vi "Compare ni-xnet port with monitoring port.vi"(8 "Error In":errorcluster, 10 "NI-XNET Port Item Ref In":T1 format="%.0x", 11 "CD Port Item Ref In":T1 format="%.0x") -> (0 "Error Out":errorcluster, 2 "NI-XNET Port Item Ref Out":T1 format="%.0x", 3 "CD Port Item Ref Out":T1=18446744073709551615 format="%.0x")   [LabVIEW 2018, in "NI-XNET Monitor System Explorer.lvlib"]
uses:
  NI-XNET Monitor System Explorer.lvlib
  <vilib>/NI Veristand/Custom Device API/Custom Device Item Ref.ctl
  Shared/Constants.vi
  <vilib>/NI Veristand/Custom Device API/Get Item Property (Boolean).vi
  <vilib>/NI Veristand/Custom Device API/Get Item Property (String).vi
  <vilib>/NI Veristand/Custom Device API/Set Item Property (String).vi
  <vilib>/NI Veristand/Custom Device API/Custom Device API.lvlib
  Shared/NI-XNET Monitor Shared.lvlib
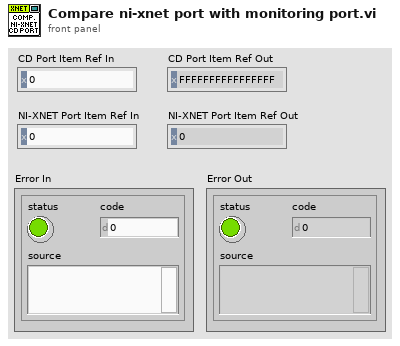
[diagram p1: front panel]
types:
  T1 = typedef "Custom Device API.lvlib/Custom Device Item Ref.ctl" = u64
  T2 = typedef "Custom Device API.lvlib/Custom Device Item Info.ctl" = cluster{"Name":string, "Is Channel":bool, "GUID":string, "Is Waveform":bool}
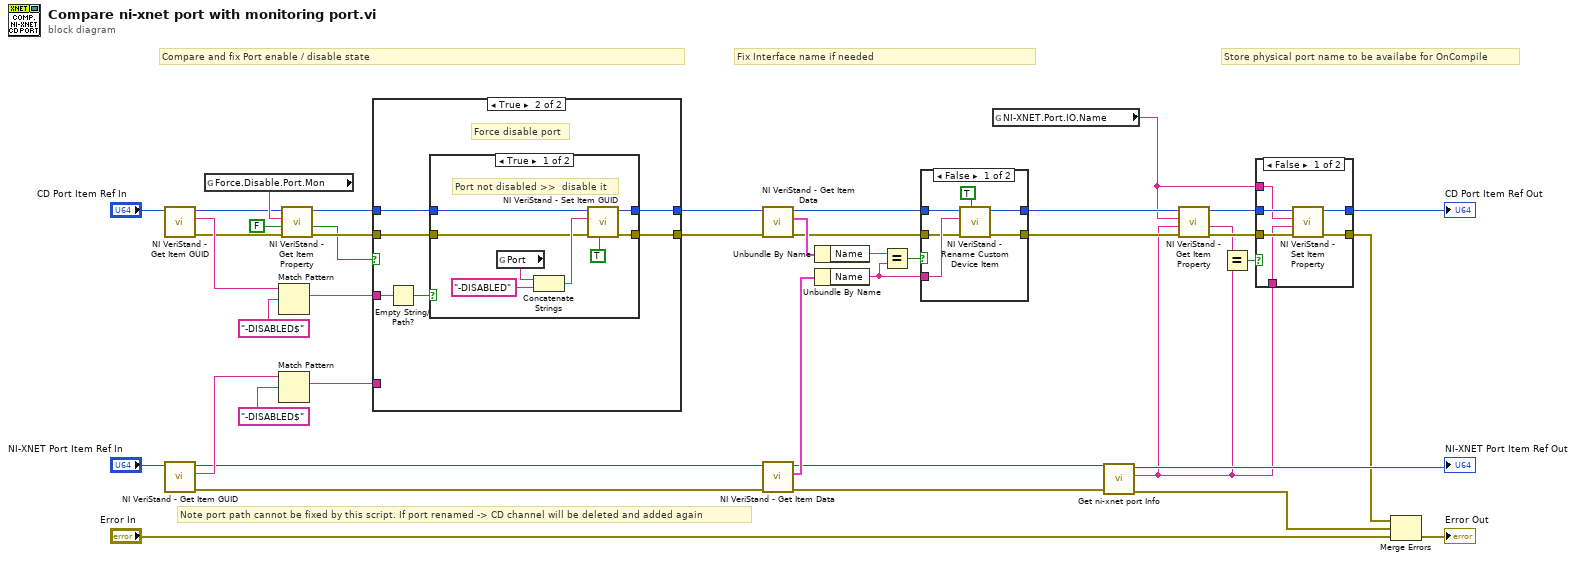
[diagram p0: block diagram]
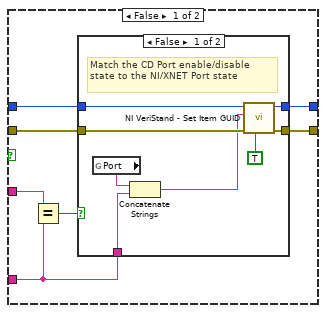
[diagram p4: hidden frame]
diagram:
  # "Note port path cannot be fixed by this script. If port renamed -> CD channel will be deleted and added again"
  # "Store physical port name to be availabe for OnCompile"
  # "Fix Interface name if needed"
  # "Compare and fix Port enable / disable state"
  n1 = call <vilib>:"NI VeriStand - Get Item GUID.vi"("Item Ref in"="CD Port Item Ref In") -> ("error out"=w33:errorcluster, "GUID"=w34:string, "Item Ref out"=w35:T1)  [unwired: 8 in]
  n2 = call <vilib>:"NI VeriStand - Get Item GUID.vi"("Item Ref in"="NI-XNET Port Item Ref In") -> ("error out"=w15:errorcluster, "GUID"=w32:string, "Item Ref out"=w31:T1)  [unwired: 8 in]
  n3 = global read "Constants.vi" "Force.Disable.Port.Mon"() -> (w39:string)
  n4 = Match Pattern(string=w34, regular expression="-DISABLED$") -> (match substring=w19:string)  [unwired: 1 in, 3 out]
  n5 = Match Pattern(string=w32, regular expression="-DISABLED$") -> (match substring=w20:string)  [unwired: 1 in, 3 out]
  n6 = call-poly <vilib>:"NI VeriStand - Get Item Property.vi"("error in (no error)"=w33, "Default Value"=FALSE, "Property Name"=w39, "Item Ref in"=w35) -> ("error out"=w36:errorcluster, "Value"=w16:bool, "Item Ref out"=w37:T1)  [unwired: 4 in, 1 out]
  n7 = case shown="True" w16 {
    tunnel: w37 -> [w46 w64]
    tunnel: w36 -> [w44 w62]
    tunnel: w20 -> [w49 _]
    tunnel: [w47 w65] -> w18
    tunnel: [w45 w63] -> w24
    tunnel: w19 -> [w48 w60]
    frame False {
      n8 = Equal?(x=w48, y=w49) -> (x = y?=w43:bool)
      n9 = case shown="False" w43 {
        tunnel: w49 -> [w56 _]
        tunnel: [w55 w59] -> w47
        tunnel: w46 -> [w53 w59]
        tunnel: [w54 w58] -> w45
        tunnel: w44 -> [w52 w58]
        frame False {
          # "Match the CD Port enable/disable state to the NI/XNET Port state"
          n10 = global read "Constants.vi" "Port"() -> (w57:string)
          n11 = Concatenate Strings(w57, w56) -> (w51:string)
          n12 = call <vilib>:"NI VeriStand - Set Item GUID.vi"("Refresh System Explorer Tree? (F)"=TRUE, "error in (no error)"=w52, "GUID"=w51, "Item Ref in"=w53) -> ("error out"=w54:errorcluster, "Item Ref out"=w55:T1)  [unwired: 6 in]
        }
        frame True {
          # "CD Port enable/disable state matches the NI/XNET Port state"
        }
      }
    }
    frame True {
      # "Force disable port"
      n13 = Empty String/Path?(string/path=w60) -> (empty?=w61:bool)
      n14 = case shown="True" w61 {
        tunnel: [w70 w75] -> w65
        tunnel: w64 -> [w71 w75]
        tunnel: [w69 w74] -> w63
        tunnel: w62 -> [w67 w74]
        frame True {
          # "Port not disabled >>  disable it"
          n15 = global read "Constants.vi" "Port"() -> (w73:string)
          n16 = Concatenate Strings(w73, "-DISABLED" ("string")) -> (w68:string)
          n17 = call <vilib>:"NI VeriStand - Set Item GUID.vi"("Refresh System Explorer Tree? (F)"=TRUE, "error in (no error)"=w67, "GUID"=w68, "Item Ref in"=w71) -> ("error out"=w69:errorcluster, "Item Ref out"=w70:T1)  [unwired: 6 in]
        }
        frame False {
          # "Port  disabled >>  do nothing"
        }
      }
    }
  }
  n18 = call <vilib>:"NI VeriStand - Get Item Data.vi"("error in (no error)"=w24, "Item Ref in"=w18) -> ("error out"=w25:errorcluster, "Item Info"=w30:T2, "Item Ref out"=w28:T1)  [unwired: 6 in, 1 out]
  n19 = call <vilib>:"NI VeriStand - Get Item Data.vi"("error in (no error)"=w15, "Item Ref in"=w31) -> ("error out"=w14:errorcluster, "Item Info"=w29:T2, "Item Ref out"=w10:T1)  [unwired: 6 in, 1 out]
  n20 = Unbundle By Name(w30) -> ("Name"=w21:string)
  n21 = Unbundle By Name(w29) -> ("Name"=w26:string)
  n22 = Equal?(x=w21, y=w26) -> (x = y?=w27:bool)
  n23 = case shown="False" w27 {
    tunnel: w28 -> [w81 w83]
    tunnel: [w80 w83] -> w8
    tunnel: w26 -> [w79 _]
    tunnel: w25 -> [w78 w82]
    tunnel: [w76 w82] -> w6
    frame False {
      n24 = call <vilib>:"NI VeriStand - Rename Custom Device Item.vi"("Force Rename (F)"=TRUE, "error in (no error)"=w78, "New Name"=w79, "Item Ref in"=w81) -> ("error out"=w76:errorcluster, "Item Ref out"=w80:T1)  [unwired: 6 out]
    }
    frame True {
    }
  }
  n25 = global read "Constants.vi" "NI-XNET.Port.IO.Name"() -> (w4:string)
  n26 = call "Get ni-xnet port Info.vi"("Error In"=w14, "NI-XNET Port Item Ref in"=w10) -> ("Error Out"=w11:errorcluster, "NI-XNET Port Name"=w2:string, "NI-XNET Port Item Ref out"=→"NI-XNET Port Item Ref Out":T1)  [unwired: 5 in, 2 out]
  n27 = call-poly <vilib>:"NI VeriStand - Get Item Property.vi"("error in (no error)"=w6, "Default Value"=w2, "Property Name"=w4, "Item Ref in"=w8) -> ("error out"=w5:errorcluster, "Value"=w3:string, "Item Ref out"=w7:T1)  [unwired: 4 in, 1 out]
  n28 = Equal?(x=w3, y=w2) -> (x = y?=w1:bool)
  n29 = case shown="False" w1 {
    tunnel: [w89 w91] -> w23
    tunnel: [w88 w90] -> w12
    tunnel: w7 -> [w87 w91]
    tunnel: w5 -> [w86 w90]
    tunnel: w4 -> [w85 _]
    tunnel: w2 -> [w84 _]
    frame False {
      n30 = call-poly <vilib>:"NI VeriStand - Set Item Property.vi"("error in (no error)"=w86, "Value"=w84, "Property Name"=w85, "Item Ref in"=w87) -> ("error out"=w88:errorcluster, "Item Ref out"=w89:T1)  [unwired: 5 in, 1 out]
    }
    frame True {
    }
  }
  "CD Port Item Ref Out" <- w23
  n31 = Merge Errors(w12, w11, "Error In") -> (→"Error Out":errorcluster)
